vi "Test_tcp_server.vi"(5 "timeout":i32=1000, 6 "value":refnum<vi>[](array[refnum]), 7 "port":u16=10000, 8 "error_in":errorcluster, 11 "conn_id_in":refnum<k5>) -> (0 "error_out":errorcluster, 3 "conn_id_out":refnum<k5>, 4 "status":string)   [LabVIEW 2019]
panel:
  out "data_type":i16[](array[numeric])
  out "message":string
  in  "clear_error":bool=TRUE
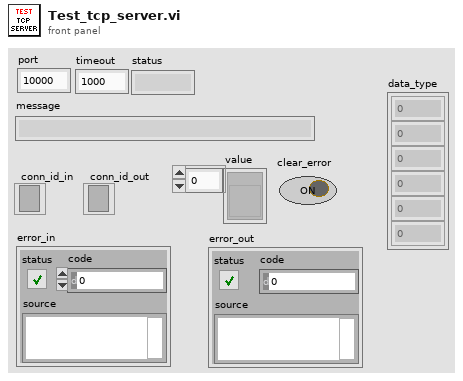
[diagram p1: front panel]
types:
  T1 = enum16{"Standard", "Buffered", "CRLF", "Immediate"}
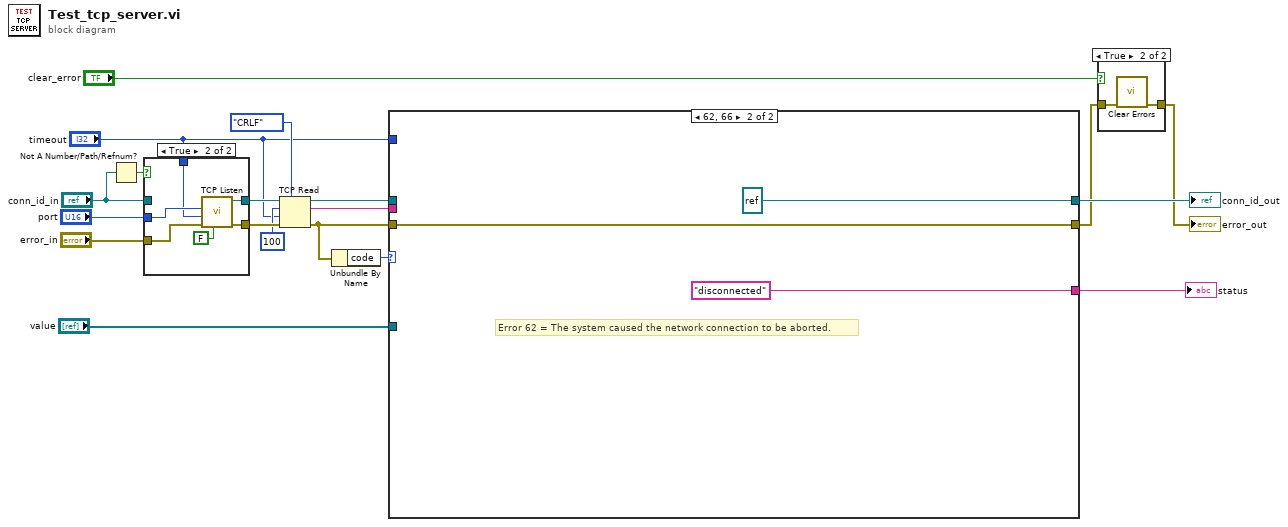
[diagram p0: block diagram]
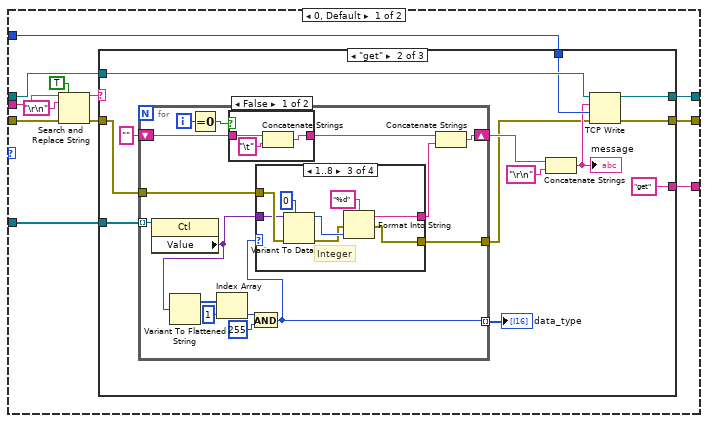
[diagram p3: hidden frame]
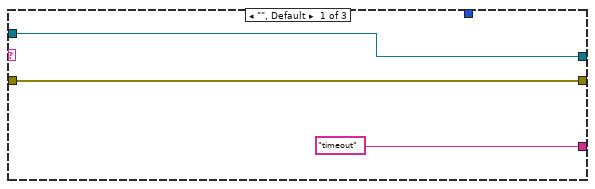
[diagram p4: hidden frame]
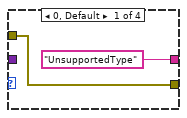
[diagram p5: hidden frame]
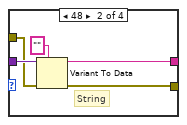
[diagram p6: hidden frame]
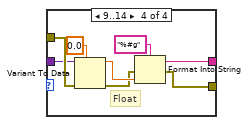
[diagram p7: hidden frame]
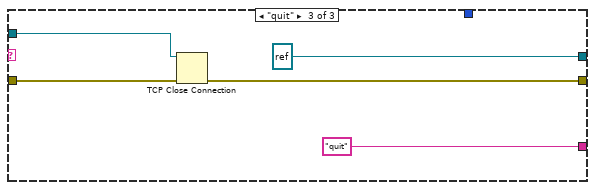
[diagram p9: hidden frame]
diagram:
  n1 = Not A Number/Path/Refnum?(number/path/refnum="conn_id_in") -> (NaN/Path/Refnum?=w19:bool)
  n2 = case shown="True" w19 {
    tunnel: [w21 w27] -> w16
    tunnel: "conn_id_in" -> [w21 _]
    tunnel: "port" -> [_ w26]
    tunnel: "timeout" -> [_ w25]
    tunnel: [w20 w23] -> w14
    tunnel: "error_in" -> [w20 w22]
    frame False {
    }
    frame True {
      n3 = call <vilib>:"TCP Listen.vi"("resolve remote address (T)"=FALSE, "error in (no error)"=w22, "timeout ms (wait forever: -1)"=w25, "port"=w26) -> ("error out"=w23:errorcluster, "connection ID"=w27:refnum<k5>)  [unwired: 3 in, 3 out]
    }
  }
  n4 = TCP Read(connection ID=w16, bytes to read=100, error in (no error)=w14, 7:T1."CRLF" ("mode (standard)"), 9:"timeout") -> (connection ID out=w10:refnum<k5>, data out=w11:string, error out=w6:errorcluster)
  n5 = Unbundle By Name(w6) -> ("code"=w5:i32)
  n6 = case shown="62, 66" w5 {
    tunnel: w11 -> [w39 _]
    tunnel: w10 -> [w35 _]
    tunnel: [w33 w104] -> w3
    tunnel: "timeout" -> [w32 _]
    tunnel: [w31 refnum<k5> refnum ("conn_id 2")] -> w8
    tunnel: [w30 "disconnected"] -> w7
    tunnel: w6 -> [w29 w104]
    tunnel: "value" -> [w28 _]
    frame 0, Default {
      n7 = Search and Replace String(replace all?=TRUE ("replace all? (F)"), input string=w39, search string="\r\n", error in=w29) -> (result string=w36:string, error out=w34:errorcluster)  [unwired: 4 in, 2 out]
      n8 = case shown="\"get\"" w36 {
        tunnel: w35 -> [w42 w54 w102]
        tunnel: w34 -> [w41 w45 w101]
        tunnel: [w42 w53 refnum<k5> refnum ("conn_id 2")] -> w31
        tunnel: [w41 w55 w99] -> w33
        tunnel: w32 -> [_ w52 _]
        tunnel: ["timeout" "get" "quit"] -> w30
        tunnel: w28 -> [_ w50 _]
        frame "", Default {
        }
        frame "get" {
          n9 = for {
            tunnel: w50 -> [w70] mode=indexing
            shift-right: [w65] -> w48
            shift-left: "" -> [w67]
            tunnel: w45 -> [w63]
            tunnel: [w62] -> w44
            tunnel: [w56] -> w43 mode=indexing
            i -> [w69]
            n10 = property on="Property Node" class="Ctl"(reference=w70) -> ("Value"=w57:variant)  [unwired: 1 in, 2 out]
            n11 = Variant To Flattened String(Variant=w57) -> (1:w60:i16[])  [unwired: 1 out]
            n12 = Equal To 0?(x=w69) -> (x = 0?=w68:bool)
            n13 = Index Array(array=w60, index=1) -> (element=w61:i16)
            n14 = case shown="False" w68 {
              tunnel: w67 -> [w96 w97]
              tunnel: [w94 w97] -> w66
              frame False {
                n15 = Concatenate Strings(w96, "\t" ("string")) -> (w94:string)
              }
              frame True {
              }
            }
            n16 = And(x=w61, y=i16 255) -> (x .and. y?=w56:i16)
            n17 = case shown="1..8" w56 {
              tunnel: w57 -> [_ w77 w78 w86]
              tunnel: ["UnsupportedType" w75 w82 w90] -> w64
              tunnel: w63 -> [w71 w74 w81 w89]
              tunnel: [w71 w73 w79 w87] -> w62
              frame 0, Default {
              }
              frame 48 {
                # "String"
                n18 = Variant To Data(error in=w74, type="", Variant=w77) -> (data=w75:string, error out=w73:errorcluster)
              }
              frame 1..8 {
                # "Integer"
                n19 = Variant To Data(error in=w81, type=i64 0 ("input 1"), Variant=w78) -> (data=w83:i64, error out=w80:errorcluster)
                n20 = Format Into String(format string="%d", error in=w80, w83) -> (resulting string=w82:string, error out=w79:errorcluster)  [unwired: 1 in]
              }
              frame 9..14 {
                # "Float"
                n21 = Variant To Data(error in=w89, type=0.0 ("input 1"), Variant=w86) -> (data=w91:dbl, error out=w88:errorcluster)
                n22 = Format Into String(format string="%#g", error in=w88, w91) -> (resulting string=w90:string, error out=w87:errorcluster)  [unwired: 1 in]
              }
            }
            n23 = Concatenate Strings(w66, w64) -> (w65:string)
          }
          "data_type" <- w43
          n24 = Concatenate Strings(w48, "\r\n" ("format string")) -> (w46:string)
          "message" <- w46
          n25 = TCP Write(connection ID=w54, data in=w46, error in (no error)=w44, 9:w52) -> (connection ID out=w53:refnum<k5>, error out=w55:errorcluster)  [unwired: 1 out]
        }
        frame "quit" {
          n26 = TCP Close Connection(connection ID=w102, error in (no error)=w101) -> (error out=w99:errorcluster)  [unwired: 1 in, 1 out]
        }
      }
    }
    frame 62, 66 {
      # "Error 62 = The system caused the network connection to be aborted."
    }
  }
  "status" <- w7
  "conn_id_out" <- w8
  n27 = case shown="True" "clear_error" {
    tunnel: w3 -> [w106 w108]
    tunnel: [w106 w107] -> w2
    frame False {
    }
    frame True {
      n28 = call <vilib>:"Clear Errors.vi"("error in (no error)"=w108) -> ("error out"=w107:errorcluster)  [unwired: 5 in, 1 out]
    }
  }
  "error_out" <- w2
